vi "While Loop Temp Converter Repeating.vi"() -> ()   [LabVIEW 2019]
panel:
  in  "Push the button to stop the program":bool
  in  "Celsius":dbl(slide) scale=0.0..100.0
  out "Kelvin":dbl(slide) scale=273.0..373.0
  out "Fahrenheit":dbl(slide) scale=0.0..212.0
  # "Challenge:\nCreate a temperature converter that converts  a temperature in degrees Celsius to degrees Kelvin and degrees Fahrenheit. Display each temperature on an appropriately scaled thermometer. Whenever the Celsius slider is moved, the other two sliders adjust as well."
  # "Try it: Run the program and change the Celsius temperature."
  # "You will probably need:\nWhile loops, indicators and controls, numeric functions"
  # "Open the block diagram to see a possible solution."
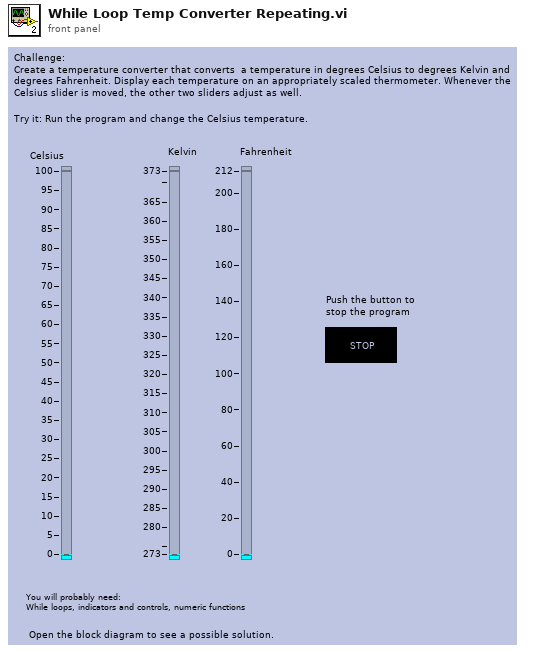
[diagram p1: front panel]
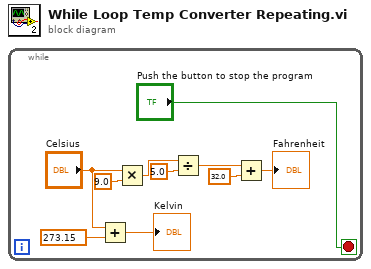
[diagram p0: block diagram]
diagram:
  n1 = while {
    stop <- "Push the button to stop the program" stop-if-true
    n2 = Add(x="Celsius", y=273.15) -> (x+y=→"Kelvin":dbl)
    n3 = Multiply(x="Celsius", y=9.0) -> (x*y=w7:dbl)
    n4 = Divide(x=w7, y=5.0) -> (x/y=w6:dbl)
    n5 = Add(x=w6, y=32.0) -> (x+y=→"Fahrenheit":dbl)
  }
